vi "Exit Event Structure.vi"(0 "Diagram in":refnum<vi>, 5 "Outputs":refnum<vi>[][](array[refnum]), 7 "Event Data Out Names":string[](array[string]), 9 "Event Data out":refnum<vi>[](array[refnum]), 11 "error in (no error)":errorcluster) -> (4 "Diagram out":refnum<vi>, 6 "Outputs":refnum<vi>[](array[refnum]), 8 "Dynamic Event Registration out":refnum<vi>, 15 "error out":errorcluster)   [LabVIEW 2015, in "Scripting.lvlib"]
doc: "Exits the Event Structure that owns <B>Diagram in</B>, supplying the structure's owning diagram at <B>Diagram out</B>.\n\n<B>Event Data Out Names</B> are the names of the desired Event Data out elements of the current frame.\n\n<B>Event Data Out<B> is an array of terminals to wire to the configured Event Data out terminals."
uses:
  Scripting.lvlib
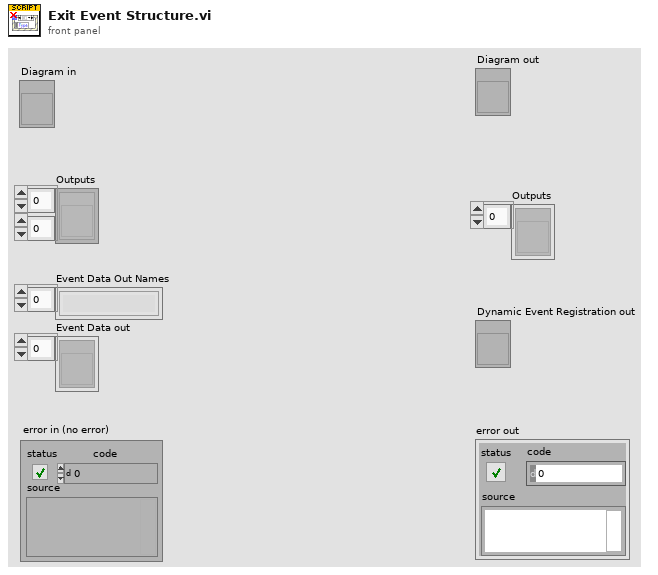
[diagram p1: front panel]
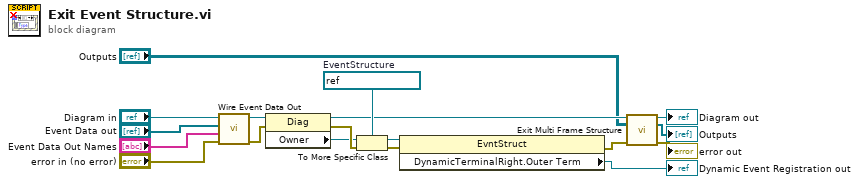
[diagram p0: block diagram]
diagram:
  w18 = refnum<vi> refnum  # EventStructure
  n1 = call "Wire Event Data Out.vi"("error in (no error)"="error in (no error)", "Event Data Names"="Event Data Out Names", "Event Data"="Event Data out", "Diagram in"="Diagram in") -> ("error out"=w11:errorcluster, "Diagram out"=w9:refnum<vi>)  [unwired: 6 in]
  n2 = property class="Diag"(reference=w9, error in=w11) -> (reference out=w7:refnum<vi>, error out=w10:errorcluster, "Owner"=w8:refnum<vi>)
  n3 = To More Specific Class(target class=w18, reference=w8, error in=w10) -> (specific class reference=w15:refnum<vi>, error out=w14:errorcluster)
  n4 = property class="EvntStruct"(reference=w15, error in=w14) -> (error out=w5:errorcluster, "DynamicTerminalRight.Outer Term"=→"Dynamic Event Registration out":refnum<vi>)  [unwired: 1 out]
  n5 = call "Exit Multi Frame Structure.vi"("Diagram in"=w7, "Outputs"="Outputs", "error in (no error)"=w5) -> ("Diagram out"=→"Diagram out":refnum<vi>, "Outputs"=→"Outputs":refnum<vi>[], "error out"=→"error out":errorcluster)  [unwired: 10 in]
